vi "Get Status.vi"(8 "error in (no error)":errorcluster, 11 "Reader.lvclass in":refnum<class "Reader.lvclass">) -> (0 "error out":errorcluster, 2 "Status":string, 3 "Reader.lvclass out":refnum<class "Reader.lvclass">)   [LabVIEW 2023, in "Reader.lvclass"]
uses:
  Reader.lvclass
  Reader.lvclass/Reader.ctl
  Global/File Locations.vi
  Instruments/Utility Classes/Readable/Readable.lvclass
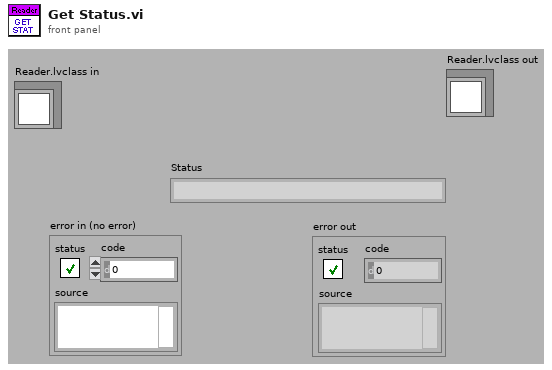
[diagram p1: front panel]
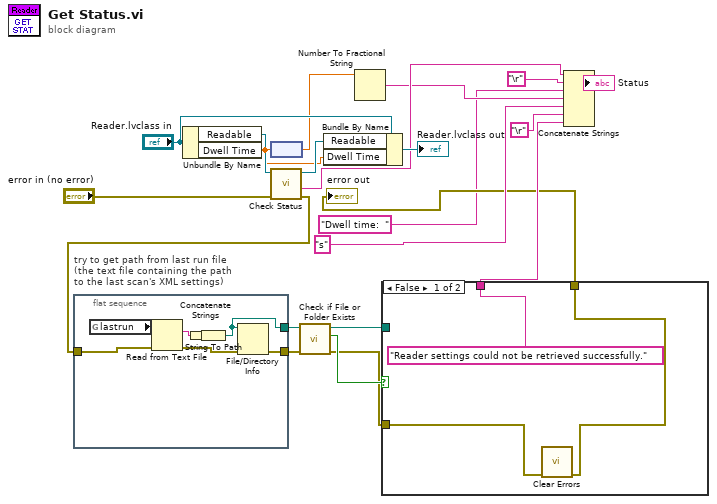
[diagram p0: block diagram]
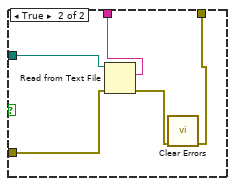
[diagram p2: hidden frame]
diagram:
  n1 = flat-sequence "try to get path from last run file\n(the text file containing the path\nto the last scan's XML settings)" {
    tunnel: [w29] -> w11
    tunnel: [w25] -> w12
    tunnel: w4 -> [w24]
    frame #0 {
      n2 = global read "File Locations.vi" "lastrun"() -> (w27:path)
      n3 = Read from Text File(file (use dialog)=w27, error in=w24) -> (text=w28:string, error out=w26:errorcluster)  [unwired: 4 out]
      n4 = Concatenate Strings(w28) -> (w23:string)
      n5 = String To Path(string=w23) -> (path=w29:path)
      n6 = File/Directory Info(path=w29, error in=w26) -> (error out=w25:errorcluster)  [unwired: 6 out]
    }
  }
  n7 = Unbundle By Name("Reader.lvclass in") -> ("Readable"=w22:refnum<class "Readable.lvclass">, "Dwell Time"=w13:dbl[unit])
  n8 = node(w13) -> (w16:dbl)
  n9 = call-dynamic "Check Status.vi"("error in (no error)"="error in (no error)", "Instrument in"=w22) -> ("error out"=w4:errorcluster, "Status"=w18:string, "Instrument out"=w20:refnum<class "Readable.lvclass">)  [unwired: 6 in, 1 out]
  n10 = call <vilib>:"Check if File or Folder Exists.vi"("error in (no error)"=w12, "path"=w11) -> ("error out"=w9:errorcluster, "file or folder exists?"=w10:bool, "dup path"=w8:path)  [unwired: 7 in]
  n11 = Bundle By Name(cluster="Reader.lvclass in", "Readable"=w20, "Dwell Time"=w13) -> (→"Reader.lvclass out":refnum<class "Reader.lvclass">)
  n12 = Number To Fractional String(number=w16) -> (F-format string=w15:string)  [unwired: 3 in]
  n13 = case shown="False" w10 {
    tunnel: w9 -> [w31 w36]
    tunnel: w8 -> [_ w37]
    tunnel: ["Reader settings could not be retrieved successfully." w35] -> w6
    tunnel: [w30 w33] -> w3
    frame False {
      n14 = call <vilib>:"Clear Errors.vi"("error in (no error)"=w31) -> ("error out"=w30:errorcluster)  [unwired: 5 in, 1 out]
    }
    frame True {
      n15 = Read from Text File(file (use dialog)=w37, error in=w36) -> (text=w35:string, error out=w34:errorcluster)  [unwired: 2 in, 2 out]
      n16 = call <vilib>:"Clear Errors.vi"("error in (no error)"=w34) -> ("error out"=w33:errorcluster)  [unwired: 5 in, 1 out]
    }
  }
  "error out" <- w3
  n17 = Concatenate Strings(w18, "\r", "Dwell time:  ", w15, "s", "\r", w6) -> (→"Status":string)
